vi "zmq_send.vi"(0 "error in":errorcluster, 2 "data":string, 3 "socket in":refnum<class "zmq_socket.lvclass">, 4 "more? (F)":bool) -> (5 "error out":errorcluster, 8 "socket out":refnum<class "zmq_socket.lvclass">)   [LabVIEW 2019, in "zeromq.lvlib" / "zmq_socket.lvclass"]
doc: "Add the binary string <b>data</b> (the NULL value \\0 is permitted) to the output queue of the socket <b>socket in</b>.\n\nIf <b>no block?</b> is True, the function returns immediately regardless of whether the message entered the queue successfully (not recommended).\n\nIf this message is part of a larger multi-component message and there are more parts to follow, then set <b>more?</b> to True.\n\nNote that when this call returns the message will likely <b>not have been sent yet</b> as it has only been placed in the queue for sending.\n\nDetailed API documentation: http://api.zeromq.org/3-2:zmq-send"
uses:
  zmq_socket.lvclass
  zmq_socket.lvclass/zmq_socket.ctl
  <vilib>/Utility/error.llb/Error Cluster From Error Code.vi
  zeromq.lvlib
panel:
  # "ØMQ"
  # "labview"
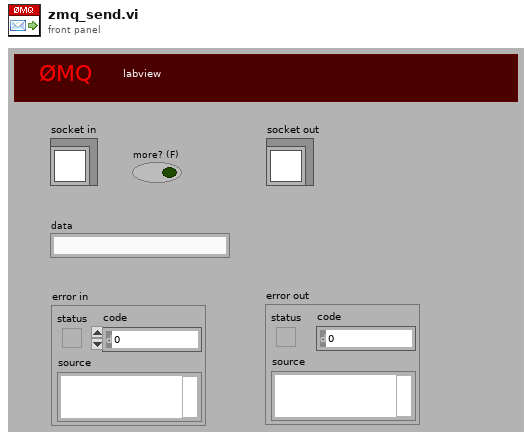
[diagram p1: front panel]
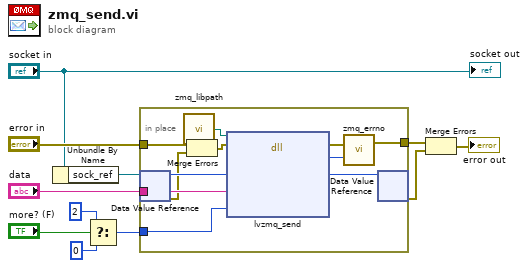
[diagram p0: block diagram]
diagram:
  n1 = Unbundle By Name("socket in") -> ("sock_ref"=w3:refnum<data-value>)
  n2 = Select(t=2 ("flags"), s="more? (F)", f=0 ("flags")) -> (s? t:f=w5:i32)
  n3 = in-place {
    in-place-border: "error in" -> [w22]
    in-place-border: "data" -> [w21]
    in-place-border: [w18] -> w9
    in-place-border: w5 -> [w17]
    n4 = in-place-dvr #1(w3) -> (w16:u64, w12:errorcluster)
    n5 = call "zmq_libpath.vi"() -> ("path"=w14:path)
    n6 = Merge Errors(w22, w12) -> (w13:errorcluster)
    n7 = dll-call lib="?" fn="lvzmq_send" ("zmq_labview.dll:lvzmq_socket")(path in=w14, error in=w13, "sock_obj"=w16, "data"=w21, "flags"=w17) -> (error out=w20:errorcluster, "return type"=w19:i32, "sock_obj"=w15:u64)  [unwired: 3 in, 1 out]
    n8 = call "zmq_errno.vi"("retval"=w19, "error in"=w20) -> ("error out"=w18:errorcluster)  [unwired: 1 out]
    n9 = in-place-dvr #1(w15) -> (w1:errorcluster)  [unwired: 1 out]
  }
  n10 = Merge Errors(w9, w1) -> (→"error out":errorcluster)
  "socket out" <- "socket in"
